vi "Find all Classes in LVProj.vi"(8 "error in (no error)":errorcluster, 11 "Project Path":path) -> (0 "error out":errorcluster, 3 "Class Paths":path[](array[path]))   [LabVIEW 2020, in "Test Finder.lvclass"]
uses:
  Test Finder.lvclass
  Test Finder.lvclass/Test Finder.ctl
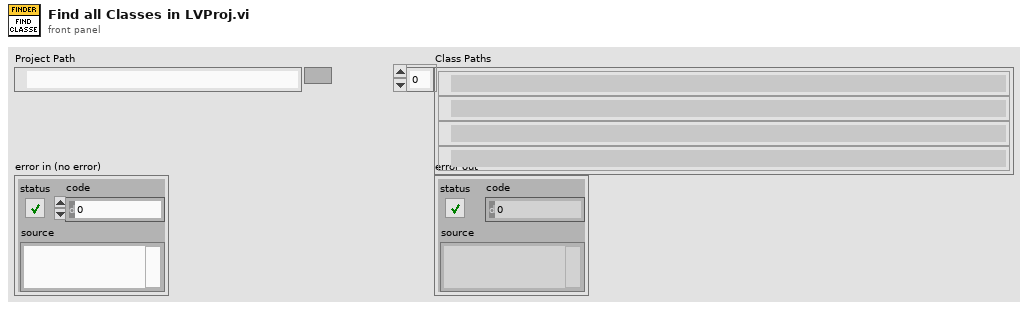
[diagram p1: front panel]
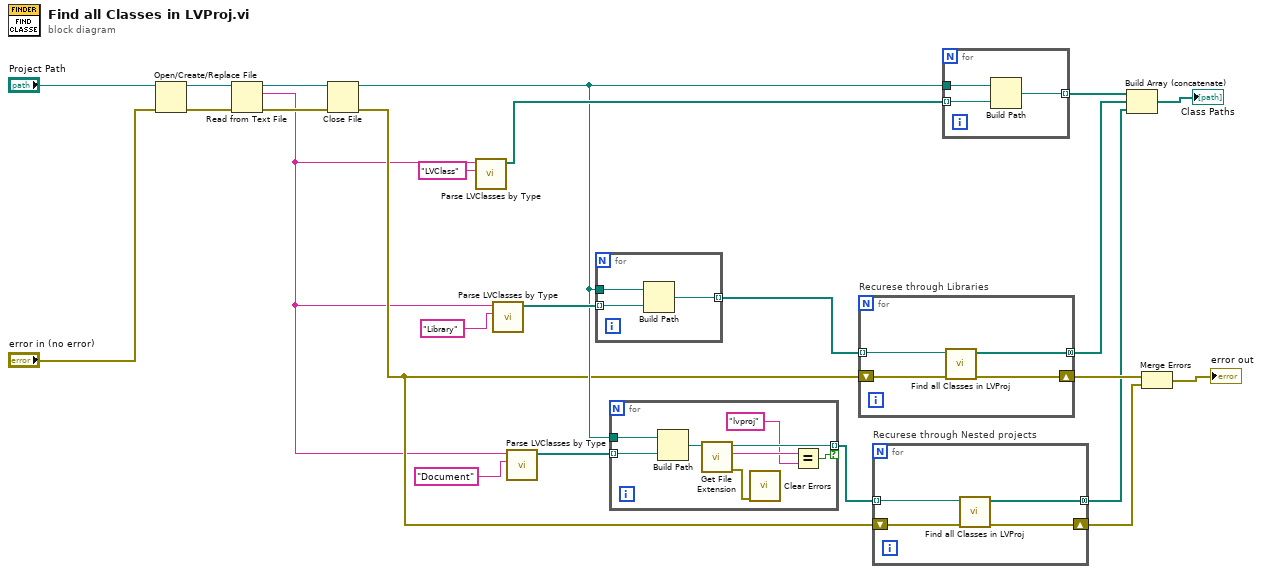
[diagram p0: block diagram]
diagram:
  n1 = Open/Create/Replace File(file path (use dialog)="Project Path", error in="error in (no error)") -> (refnum out=w22:refnum<file>, error out=w21:errorcluster)  [unwired: 4 in, 1 out]
  n2 = Read from Text File(file (use dialog)=w22, error in=w21) -> (refnum out=w20:refnum<file>, text=w1:string, error out=w19:errorcluster)  [unwired: 2 in, 1 out]
  n3 = Close File(refnum=w20, error in=w19) -> (path=w6:path, error out=w5:errorcluster)
  n4 = call "Parse LVClasses by Type.vi"("Type"="LVClass", "Input"=w1) -> ("Relative Paths"=w18:path[])  [unwired: 9 in]
  n5 = call "Parse LVClasses by Type.vi"("Type"="Library", "Input"=w1) -> ("Relative Paths"=w14:path[])  [unwired: 9 in]
  n6 = call "Parse LVClasses by Type.vi"("Type"="Document", "Input"=w1) -> ("Relative Paths"=w8:path[])  [unwired: 9 in]
  n7 = for {
    tunnel: w6 -> [w27]
    tunnel: w14 -> [w26] mode=indexing
    tunnel: [w25] -> w12 mode=indexing
    n8 = Build Path(base path=w27, name or relative path=w26) -> (appended path=w25:path)
  }
  n9 = for {
    tunnel: w6 -> [w35]
    tunnel: w8 -> [w34] mode=indexing
    tunnel: [w32] -> w9 mode=indexing if=w28
    n10 = Build Path(base path=w35, name or relative path=w34) -> (appended path=w33:path)
    n11 = call <vilib>:"Get File Extension.vi"("file"=w33) -> ("error out"=w29:errorcluster, "lowercase file extension"=w31:string, "dup file"=w32:path)  [unwired: 6 in, 2 out]
    n12 = call <vilib>:"Clear Errors.vi"("error in (no error)"=w29) -> ()  [unwired: 5 in, 2 out]
    n13 = Equal?(x=w31, y="lvproj") -> (x = y?=w28:bool)
  }
  n14 = for "Recurese through Libraries" {
    tunnel: w12 -> [w37] mode=indexing
    shift-right: [w38] -> w13
    shift-left: w5 -> [w39]
    tunnel: [w36] -> w11 mode=concatenating
    n15 = call "Find all Classes in LVProj.vi"("error in (no error)"=w39, "Project Path"=w37) -> ("error out"=w38:errorcluster, "Class Paths"=w36:path[])  [unwired: 8 in]
  }
  n16 = for "Recurese through Nested projects" {
    tunnel: w9 -> [w41] mode=indexing
    shift-right: [w42] -> w3
    shift-left: w5 -> [w43]
    tunnel: [w40] -> w2 mode=concatenating
    n17 = call "Find all Classes in LVProj.vi"("error in (no error)"=w43, "Project Path"=w41) -> ("error out"=w42:errorcluster, "Class Paths"=w40:path[])  [unwired: 8 in]
  }
  n18 = for {
    tunnel: w6 -> [w46]
    tunnel: w18 -> [w45] mode=indexing
    tunnel: [w44] -> w17 mode=indexing
    n19 = Build Path(base path=w46, name or relative path=w45) -> (appended path=w44:path)
  }
  n20 = Build Array (concatenate)(w17, w11, w2) -> (→"Class Paths":path[])
  n21 = Merge Errors(w13, w3) -> (→"error out":errorcluster)
